vi "Number to Match.vi"() -> ()   [LabVIEW 2021]
panel:
  in  "stop":bool
  out "Iterations":i32
  in  "Number to Match":dbl
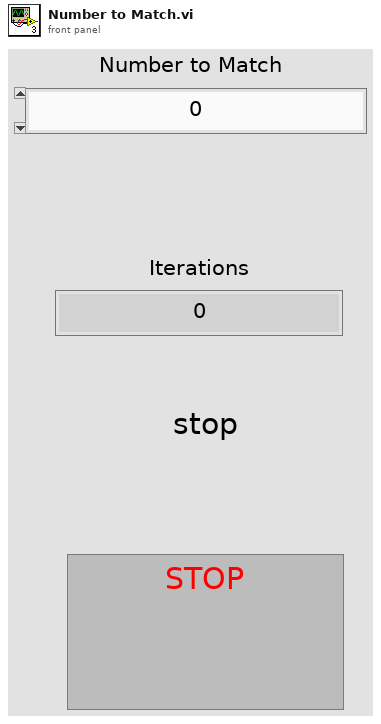
[diagram p1: front panel]
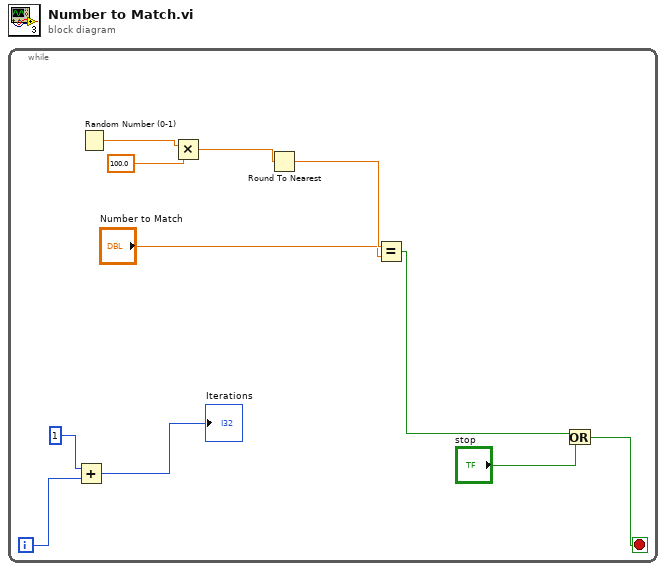
[diagram p0: block diagram]
diagram:
  n1 = while {
    i -> [w3]
    stop <- w9 stop-if-true
    n2 = Add(x=1, y=w3) -> (x+y=→"Iterations":i32)
    n3 = Random Number (0-1)() -> (number: 0 to 1=w8:dbl)
    n4 = Multiply(x=w8, y=100.0) -> (x*y=w6:dbl)
    n5 = Round To Nearest(number=w6) -> (nearest integer value=w5:dbl)
    n6 = Equal?(x=w5, y="Number to Match") -> (x = y?=w10:bool)
    n7 = Or(x=w10, y="stop") -> (x .or. y?=w9:bool)
  }
